vi "3.2 Grab FPGA Data.vi"() -> (0 "Steering Velocity":dbl, 1 "Numeric 2":dbl, 2 "Numeric":dbl, 3 "Has Refrence":bool, 4 "Steering Position":dbl, 5 "Lidar Position":dbl, 6 "Drive Velocity":dbl, 7 "Drive Position":dbl, 8 "Lidar Velocity":dbl, 9 "Has Reference":bool)   [LabVIEW 2010]
uses:
  <vilib>/rvi/interface/nirviReadWriteControl/nirviReadWriteControl.xnode
  FPGA Bitfiles/1Hindbrain.lvbitx
  1-Hindbrain.vi
  2-Low Neurons/2.1 Act Debug.ctl
  <vilib>/rvi/interface/common/niFpgaNodeNameForErrorReporting.ctl
  <vilib>/rvi/errors/niLvFpgaWhatHappensToTopLevelVI.ctl
  3.0-Global.vi
  <vilib>/Utility/error.llb/Error Cluster From Error Code.vi
  <vilib>/rvi/errors/niLvFpgaAdjustHostInterfaceError.vi
  NiFpgaLv.dll
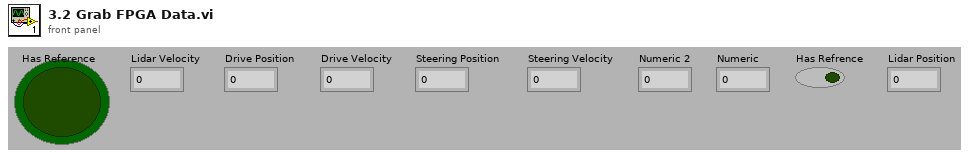
[diagram p1: front panel]
types:
  T1 = cluster{"2.1 Act Debug.Drive.Drive Position Integer":i32, "2.1 Act Debug.Steering.Steering Position Integer":i32, "2.1 Act Debug.Lidar.Lidar Position Integer":i32, "2.1 Act Debug.Drive.2.1 Drive Control Voltage":fxp<+/-,20,5>, "2.1 Act Debug.Steering.2.1  Steering Control Voltage":fxp<+/-,20,5>, "2.1 Act Debug.Drive.Motor Speed Integer":fxp<+/-,10,8>, "2.1 Act Debug.Steering.Steering V":fxp<+/-,10,8>}
  T2 = typedef "2.1 Act Debug.ctl" = cluster{"Drive":cluster{"2.1 Drive Control Voltage":fxp<+/-,20,5>, "2.1 Drive PID Output":fxp<+/-,20,5>, "2.1.1 Drive Error":fxp<+/-,18,1>, "2.1.1 Drive Error I":fxp<+/-,64,46>, "2.1.1 Drive Error D":fxp<+/-,18,1>, "Motor Speed Integer":fxp<+/-,10,8>, "Drive Position Integer":i32}, "Steering":cluster{"2.1  Steering Control Voltage":fxp<+/-,20,5>, "2.1  Steering Lead Output":fxp<+/-,20,5>, "Steering V":fxp<+/-,10,8>, "Steering Position Integer":i32, "2.1.2 sqrt(10)s+bdt":fxp<+/-,18,20>, "2.1.2 (sqrt(10)s+bdt)/(s/sqrt(10)+bdt)":fxp<+/-,20,22>, "2.1.2 s(sqrt(10)s+bdt)/(s/sqrt(10)+bdt)":fxp<+/-,20,22>}, "Lidar":cluster{"2.1  Lidar Control Voltage":fxp<+/-,20,5>, "2.1  Lidar PID Output":fxp<+/-,20,5>, "2.1.3 Lidar Error":fxp<+/-,18,1>, "2.1.3 Lidar Error I":fxp<+/-,64,46>, "2.1.3 Lidar Error D":fxp<+/-,18,1>, "Lidar Position Integer":i32, "Lidar Motor Position Integer":i32}}
  T3 = typedef "niFpgaNodeNameForErrorReporting.ctl" = enum16{"Open FPGA VI Reference", "Read/Write Control", "Invoke Method: Abort", "Invoke Method: Acknowledge IRQ", "Invoke Method: Download", "Invoke Method: FIFO.Configure", "Invoke Method: FIFO.Read", "Invoke Method: FIFO.Start", "Invoke Method: FIFO.Stop", "Invoke Method: FIFO.Write", "Invoke Method: Reset", "Invoke Method: Run", "Invoke Method: Wait on IRQ", "Close FPGA VI Reference"}
  T4 = typedef "niLvFpgaWhatHappensToTopLevelVI.ctl" = enum16{"top level VI scripted behind XNode", "top level VI inlined behind XNode"}
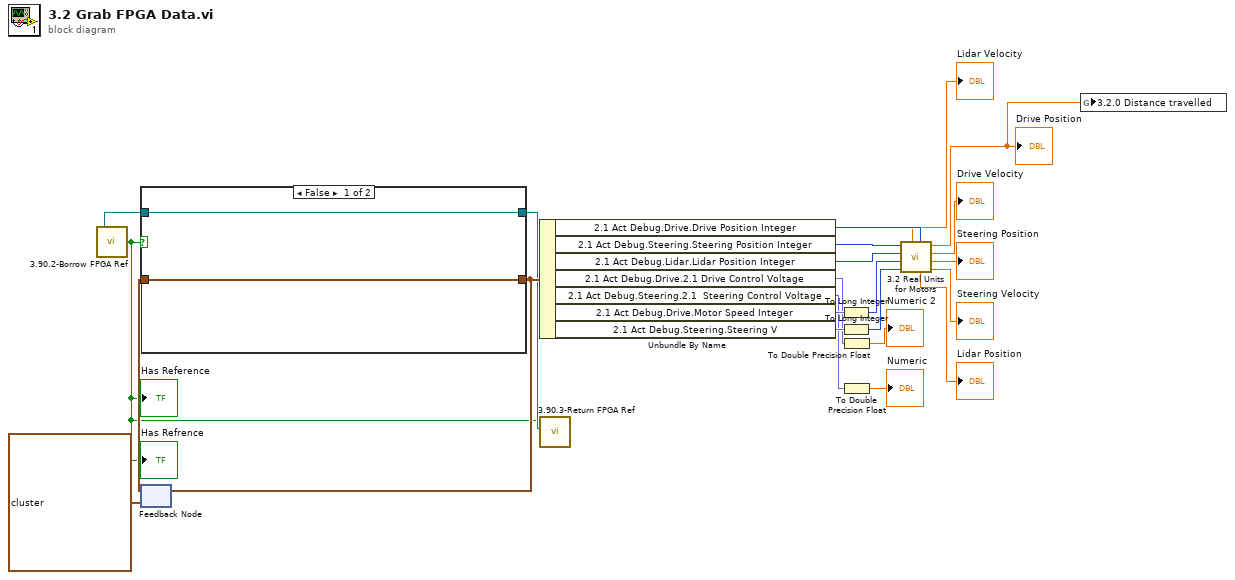
[diagram p0: block diagram]
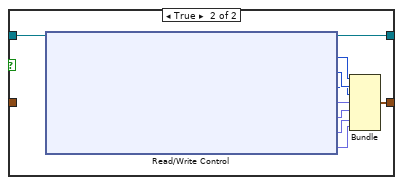
[diagram p2: hidden frame]
diagram:
  n1 = call "3.90.2-Borrow FPGA Ref.vi"() -> ("Has Refrence"=w3:bool, "Ref Out"=w4:refnum<k20>)
  "Has Reference" <- w3
  "Has Refrence" <- w3
  n2 = feedback #1(T1 {"2.1 Act Debug.Drive.Drive Position Integer"=0, "2.1 Act Debug.Steering.Steering Position Integer"=0, "2.1 Act Debug.Lidar.Lidar Position Integer"=0, "2.1 Act Debug.Drive.2.1 Drive Control Voltage"=0.0, "2.1 Act Debug.Steering.2.1  Steering Control Voltage"=0.0, "2.1 Act Debug.Drive.Motor Speed Integer"=0.0, "2.1 Act Debug.Steering.Steering V"=0.0}) -> (w15:T1)
  n3 = case shown="False" w3 {
    tunnel: w4 -> [w24 w35]
    tunnel: [w24 w34] -> w5
    tunnel: w15 -> [w25 _]
    tunnel: [w25 w26] -> w16
    frame False {
    }
    frame True {
      n4 = xnode "Read/Write Control"("FPGA VI Reference In"=w35) -> ("FPGA VI Reference Out"=w34:refnum<k20>, "2.1 Act Debug.Drive.Drive Position Integer"=w33:i32, "2.1 Act Debug.Steering.Steering Position Integer"=w32:i32, "2.1 Act Debug.Lidar.Lidar Position Integer"=w31:i32, "2.1 Act Debug.Drive.2.1 Drive Control Voltage"=w30:fxp<+/-,20,5>, "2.1 Act Debug.Steering.2.1  Steering Control Voltage"=w29:fxp<+/-,20,5>, "2.1 Act Debug.Drive.Motor Speed Integer"=w28:fxp<+/-,10,8>, "2.1 Act Debug.Steering.Steering V"=w27:fxp<+/-,10,8>)  [unwired: 1 in, 1 out]
      n5 = Bundle("2.1 Act Debug.Drive.Drive Position Integer"=w33, "2.1 Act Debug.Steering.Steering Position Integer"=w32, "2.1 Act Debug.Lidar.Lidar Position Integer"=w31, "2.1 Act Debug.Drive.2.1 Drive Control Voltage"=w30, "2.1 Act Debug.Steering.2.1  Steering Control Voltage"=w29, "2.1 Act Debug.Drive.Motor Speed Integer"=w28, "2.1 Act Debug.Steering.Steering V"=w27) -> (w26:T1)  [unwired: 1 in]
    }
  }
  n6 = feedback-in #1(w16) -> ()
  n7 = Unbundle By Name(w16) -> ("2.1 Act Debug.Drive.Drive Position Integer"=w17:i32, "2.1 Act Debug.Steering.Steering Position Integer"=w18:i32, "2.1 Act Debug.Lidar.Lidar Position Integer"=w19:i32, "2.1 Act Debug.Drive.2.1 Drive Control Voltage"=w20:fxp<+/-,20,5>, "2.1 Act Debug.Steering.2.1  Steering Control Voltage"=w21:fxp<+/-,20,5>, "2.1 Act Debug.Drive.Motor Speed Integer"=w22:fxp<+/-,10,8>, "2.1 Act Debug.Steering.Steering V"=w23:fxp<+/-,10,8>)
  n8 = call "3.90.3-Return FPGA Ref.vi"("element"=w5, "Has Refrence"=w3) -> ()  [unwired: 3 in]
  n9 = To Long Integer(number=w22) -> (32bit integer=w8:i32)
  n10 = To Long Integer(number=w23) -> (32bit integer=w9:i32)
  n11 = To Double Precision Float(number=w20) -> (double precision float=→"Numeric 2":dbl)
  n12 = To Double Precision Float(number=w21) -> (double precision float=→"Numeric":dbl)
  n13 = call "3.2 Real Units for Motors.vi"("Numeric"=w9, "Numeric 2"=w8, "2.1 Act Debug.Lidar.Lidar Position Integer"=w19, "2.1 Act Debug.Steering.Steering Position Integer"=w18, "2.1 Act Debug.Drive.Drive Position Integer"=w17) -> ("Lidar Velocity"=→"Lidar Velocity":dbl, "Lidar Position"=→"Lidar Position":dbl, "Steering Velocity"=→"Steering Velocity":dbl, "Steering Position"=→"Steering Position":dbl, "Drive Velocity"=→"Drive Velocity":dbl, "Drive Position"=w1:dbl)
  "Drive Position" <- w1
  n14 = global write "3.0-Global.vi" "3.2.0 Distance travelled"(w1) -> ()
